vi "QSM Init.vi"(11 "error in":errorcluster) -> (15 "error out":errorcluster)   [LabVIEW 2011]
uses:
  Loop ID.ctl
  QSM State List.ctl
  emi Lib/System 01/0 - General/App/Loop control 2/Private/_emi_SMLoop Register new.vi
  emi Lib/System 01/0 - General/App/Loop control/Private/_emi_GFV Loop Running.vi
  emi Lib/System 01/0 - General/App/Loop control/Private/_emi_GFV Loop Enable.vi
  emi Lib/System 01/0 - General/App/Loop control/Private/_emi_GFV Loop Linking.vi
  emi Lib/System 01/0 - General/App/Loop control 2/Private/_emi_ SMLoop Restart.vi
  emi Lib/System 01/0 - General/App/Loop control/Private/_emi_GFV stop a loop so it can reset.vi
  emi Lib/System 01/0 - General/App/Loop control 2/Private/_emi_ SMLoop Restart Counter.vi
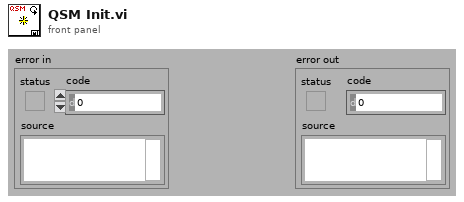
[diagram p1: front panel]
types:
  T1 = typedef "QSM State List.ctl" = enum16{"Idle", "Init <<<Start>>>", "Init Reg Controlers", "Init Stroker Ref FGV", "Init Driller Ref FGV", "Init Tractor Ref FGV", "Init All loops", "Init Mem Ctls", "Init GUI", "Init<<<End>>>", "Show options", "Options updated", "Show User Dialog", "User Updated", "Show About", "Show Help", "Debug Visibility", "End Application", "Mem Ctls", "Mem Graphs", "Post", "-------------", "Dialog Common Analog", "Chart Init", "Chart Var Selector Rings init", "Chart Read Settings from INI", "Chart Clear", "Chart Selection Changed", "Chart Time Changed", "Graph Dialog Show", "Annotation, New", "Annotation Created", "PCP CMD", "Show Welcome screen", "Dialog Tool analog", "Update PCP resistance", "Tool CMD", "Chart single autoscale", "Tool connenction state", "Show detailed view", "Sequences updated", "Show stroker wizard", "Change tool", "Reset Telemetry", "Update control units", "Stop Logging", "Start New Loggfile", "Log Init", "Copy INI files"}
  T2 = typedef "Loop ID.ctl" = enum16{"Main-QSM", "Main-Dialog", "Main-Ind Upd", "Main-Graph Upd", "Main-Debug", "Main-DebugW1", "Main-DebugW2", "Main-SE Handler", "Interface-PCP", "Interface-CANbus", "Interface-Modem", "Var Handling-Beat", "Var Handling-From PCP", "Var Handling-File storage", "Var Handling-From Simulator", "GUI-GrphW Mast", "GUI-GrphW Slav", "SIM-Tool W1", "SIM-Tool W2", "Alm-Sound", "LEIN-motor", "Tool data gatherer Qer", "Tool Data LEIN STAT2 dekoder", "Indicator Value Update", "Tool STAT2 dedicated reader", "Tool ID handler", "Detail View L1", "Detail View L2", "Main display enable view", "Sequence runner", "Voltage setpoint", "Resistance setpoint", "Stroker Wizard L1", "Stroker Wizard L2", "Alarm Handling", "Annotations Tip Strip", "Magna Interface", "Modem Status", "Var Handling - Modem Status", "Power interface detector"}
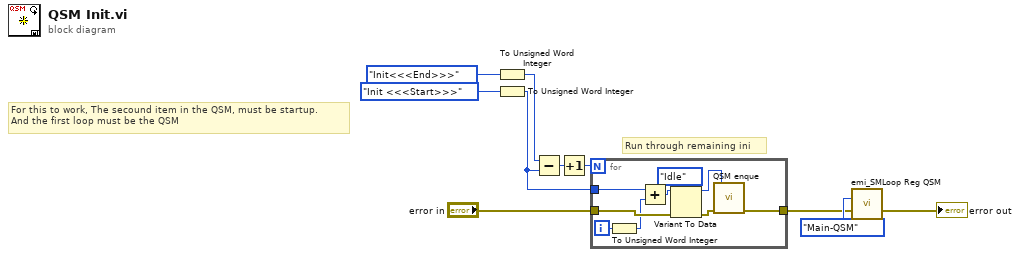
[diagram p0: block diagram]
diagram:
  # "Run through remaining ini"
  # "For this to work, The secound item in the QSM, must be startup.\nAnd the first loop must be the QSM"
  n1 = To Unsigned Word Integer(number=QSM_State_List."Init<<<End>>>" ("SMAct")) -> (unsigned 16bit integer=w8:u16)
  n2 = To Unsigned Word Integer(number=QSM_State_List."Init <<<Start>>>" ("SMAct")) -> (unsigned 16bit integer=w3:u16)
  n3 = Subtract(x=w8, y=w3) -> (x-y=w7:u16)
  n4 = Increment(x=w7) -> (x+1=w2:u16)
  n5 = for {
    N: w2 -> [_]
    tunnel: "error in" -> [w19]
    tunnel: w3 -> [w18]
    tunnel: [w12] -> w6
    i -> [w17]
    n6 = To Unsigned Word Integer(number=w17) -> (unsigned 16bit integer=w15:u16)
    n7 = Add(x=w18, y=w15) -> (x+y=w16:u16)
    n8 = Variant To Data(error in=w19, type=QSM_State_List."Idle" ("SMAct"), Variant=w16) -> (data=w11:T1, error out=w13:errorcluster)
    n9 = call "QSM enque.vi"("State"=w11, "error in"=w13) -> ("error out"=w12:errorcluster)  [unwired: 13 in]
  }
  n10 = call "emi_SMLoop Reg QSM.vi"("Loop ID"=Loop_ID."Main-QSM", "error in (no error)"=w6) -> ("error out"=→"error out":errorcluster)  [unwired: 12 in, 1 out]
